vi "Parse QD Text.vi"(11 "QD Text":string) -> ()   [LabVIEW 2020]
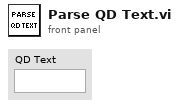
[diagram p1: front panel]
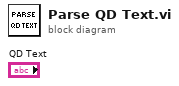
[diagram p0: block diagram]
diagram:
